vi "Feu.vi"() -> ()   [LabVIEW 2018]
uses:
  Global 1.vi
panel:
  in  "stop":bool
  out "Vert":bool
  out "Orange":bool
  out "Rouge":bool
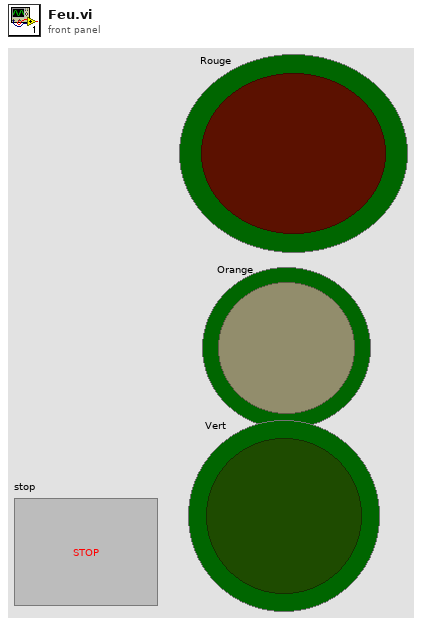
[diagram p1: front panel]
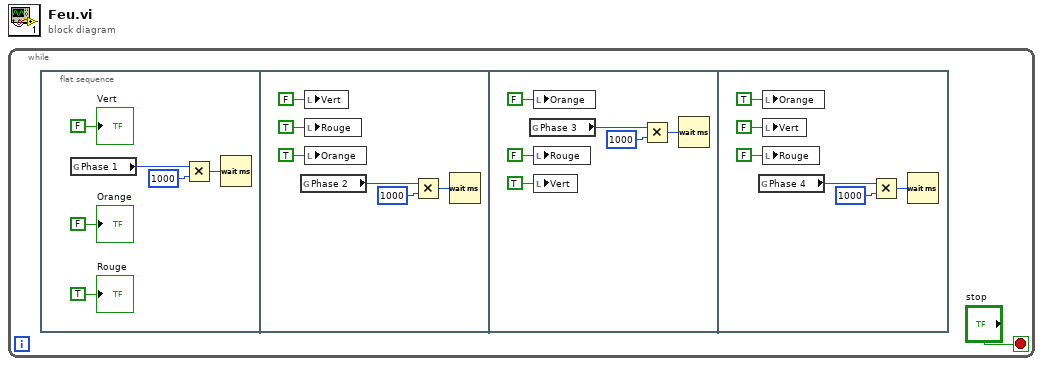
[diagram p0: block diagram]
diagram:
  n1 = while {
    stop <- "stop" stop-if-true
    n2 = flat-sequence {
      frame #0 {
        n3 = global read "Global 1.vi" "Phase 1"() -> (w2:i16)
        n4 = Multiply(x=w2, y=i16 1000) -> (x*y=w3:i16)
        n5 = Wait (ms)(milliseconds to wait=w3) -> ()  [unwired: 1 out]
        "Rouge" <- TRUE ("Boolean")
        "Orange" <- FALSE ("Boolean 2")
        "Vert" <- FALSE ("Boolean 3")
      }
      frame #1 {
        n6 = global read "Global 1.vi" "Phase 2"() -> (w8:i16)
        n7 = local write "Vert"(FALSE ("Boolean 3")) -> ()
        n8 = local write "Rouge"(TRUE ("Boolean")) -> ()
        n9 = local write "Orange"(TRUE ("Boolean 2")) -> ()
        n10 = Multiply(x=w8, y=i16 1000) -> (x*y=w9:i16)
        n11 = Wait (ms)(milliseconds to wait=w9) -> ()  [unwired: 1 out]
      }
      frame #2 {
        n12 = global read "Global 1.vi" "Phase 3"() -> (w14:i16)
        n13 = local write "Orange"(FALSE ("Boolean 2")) -> ()
        n14 = local write "Rouge"(FALSE ("Boolean")) -> ()
        n15 = local write "Vert"(TRUE ("Boolean 3")) -> ()
        n16 = Multiply(x=w14, y=i16 1000) -> (x*y=w15:i16)
        n17 = Wait (ms)(milliseconds to wait=w15) -> ()  [unwired: 1 out]
      }
      frame #3 {
        n18 = global read "Global 1.vi" "Phase 4"() -> (w20:i16)
        n19 = local write "Orange"(TRUE ("Boolean 2")) -> ()
        n20 = local write "Vert"(FALSE ("Boolean 3")) -> ()
        n21 = local write "Rouge"(FALSE ("Boolean")) -> ()
        n22 = Multiply(x=w20, y=i16 1000) -> (x*y=w21:i16)
        n23 = Wait (ms)(milliseconds to wait=w21) -> ()  [unwired: 1 out]
      }
    }
  }
